vi "Upsampling.vi"(1 "L":i32, 2 "x":cdb[](array[numeric]) format="%.2f") -> (0 "y":cdb[](array[numeric]) format="%.2f")   [LabVIEW 2011]
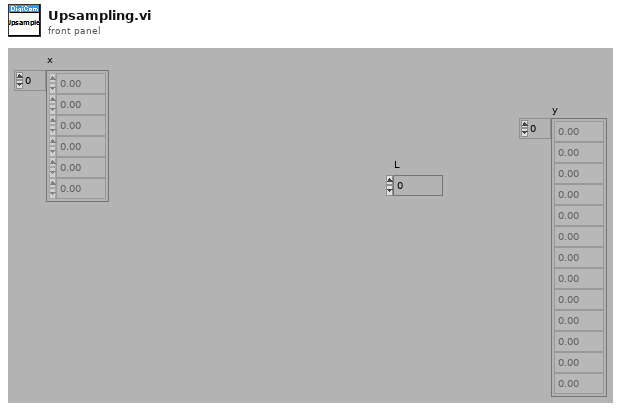
[diagram p1: front panel]
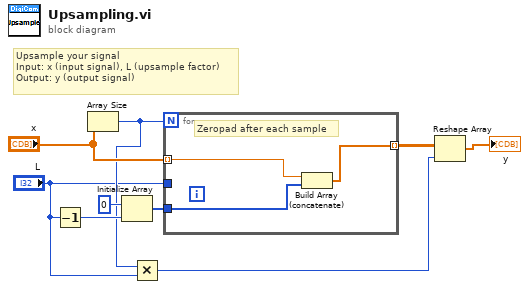
[diagram p0: block diagram]
diagram:
  # "Upsample your signal\nInput: x (input signal), L (upsample factor)\nOutput: y (output signal)"
  n1 = Decrement(x="L") -> (x-1=w6:i32)
  n2 = Array Size(array="x") -> (size(s)=w5:i32)
  n3 = Initialize Array(0, w6) -> (w8:i32[])
  n4 = Multiply(x=w5, y="L") -> (x*y=w2:i32)
  n5 = for {
    N: w5 -> [_]
    tunnel: w8 -> [w11]
    tunnel: "x" -> [w12] mode=indexing
    tunnel: [w10] -> w3 mode=indexing
    tunnel: "L" -> [_]
    # "Zeropad after each sample"
    n6 = Build Array (concatenate)(w12, w11) -> (w10:cdb[])
  }
  n7 = Reshape Array(w3, w2) -> (→"y":cdb[])
